vi "Main.vi"() -> ()   [LabVIEW 2017]
uses:
  GlobalFlash.vi
panel:
  out "?":dbl(slide) scale=0.0..100.0
  in  "Enable Alarm 7":bool=TRUE
  in  "Enable Alarm 6":bool=TRUE
  in  "Sensor 5":dbl(slide) scale=0.0..100.0
  out "Enable Alarm 5":u32(colorbox)=350218
  in  "Enable Alarm 5":bool
  in  "Sensor 4":dbl(slide) scale=0.0..100.0
  out "Enable Alarm 4":u32(colorbox)=350218
  in  "Enable Alarm 4":bool
  in  "Sensor 3":dbl(slide) scale=0.0..100.0
  out "?":u32(colorbox)=350218
  in  "Enable Alarm 3":bool
  out "?":u32(colorbox)=350218
  in  "Enable Alarm 2":bool
  in  "Sensor 2":dbl(slide) scale=0.0..100.0
  out "?":u32(colorbox)=350218
  in  "Reset1":bool
  in  "Reset2":bool
  in  "Reset3":bool
  in  "Reset4":bool
  in  "Reset5":bool
  in  "Enable Alarm 1":bool
  in  "Sensor 1":dbl(slide) scale=0.0..100.0
  # "°c"
  # "Management"
  # "Self test"
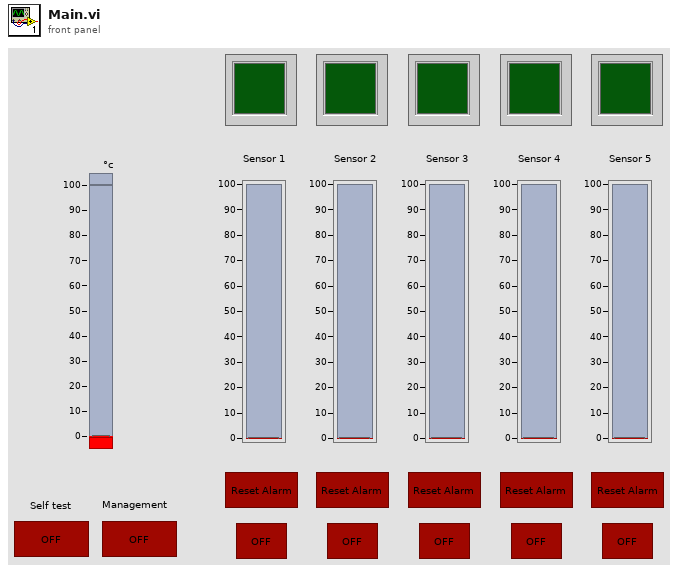
[diagram p1: front panel]
types:
  T1 = enum8{"Enabled", "Disabled", "Disabled and Grayed Out"}
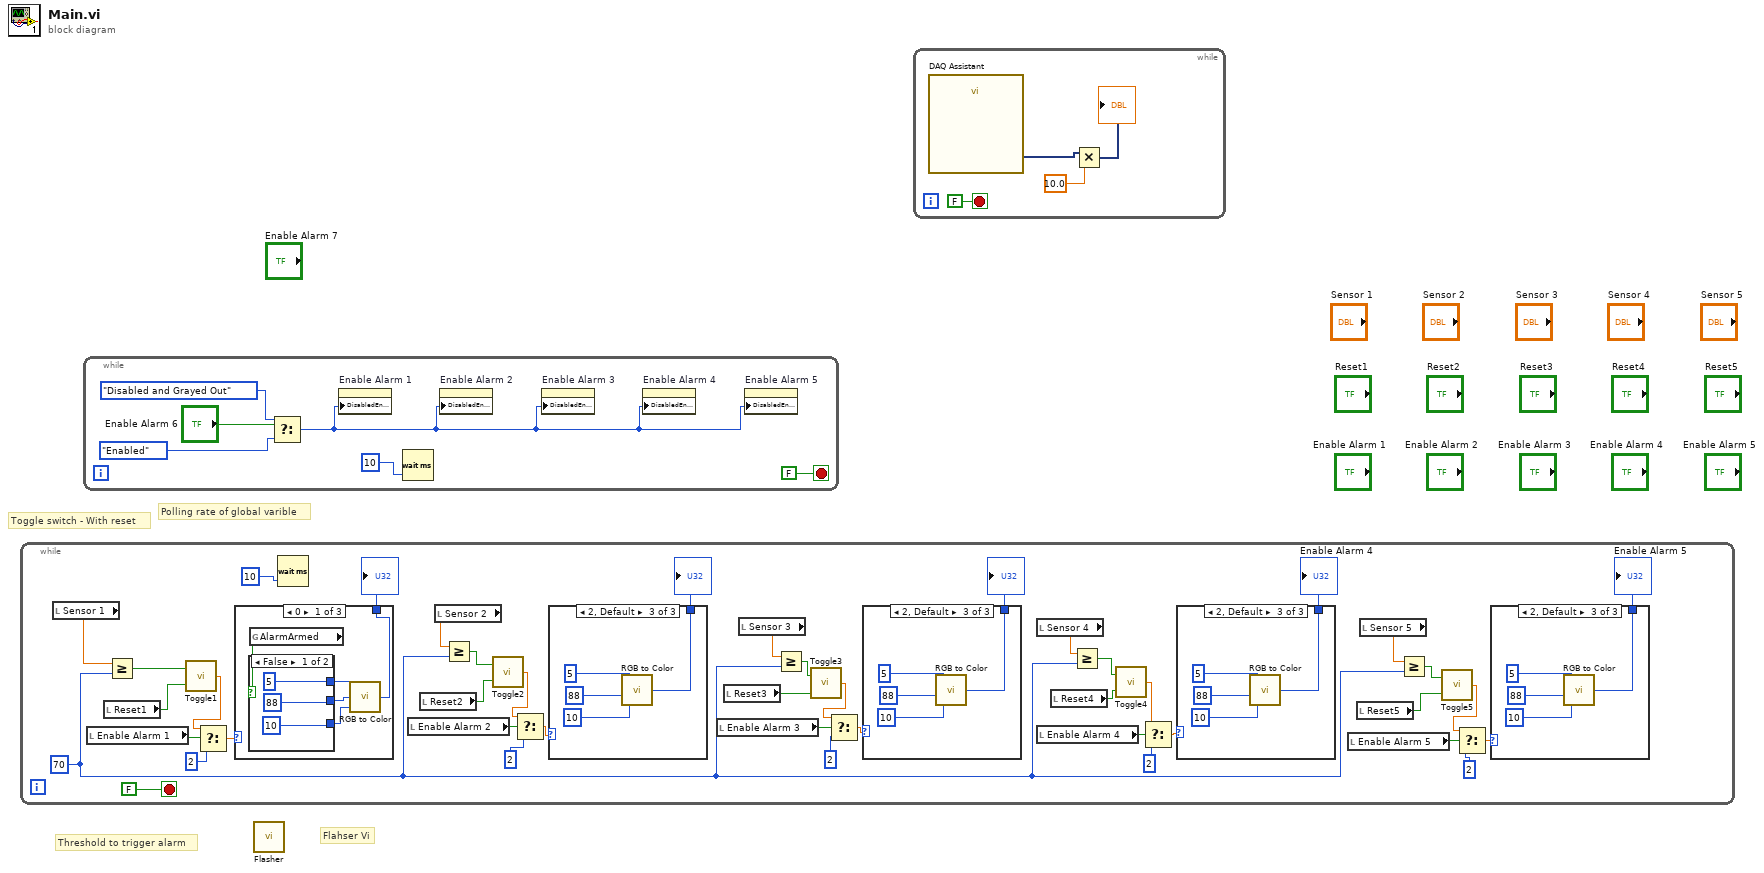
[diagram p0: block diagram]
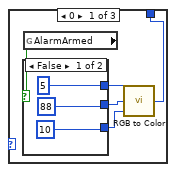
[diagram p2: hidden frame]
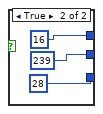
[diagram p3: hidden frame]
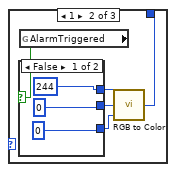
[diagram p4: hidden frame]
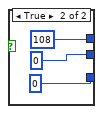
[diagram p5: hidden frame]
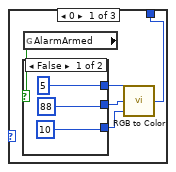
[diagram p6: hidden frame]
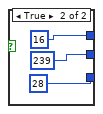
[diagram p7: hidden frame]
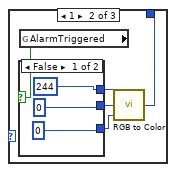
[diagram p8: hidden frame]
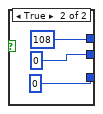
[diagram p9: hidden frame]
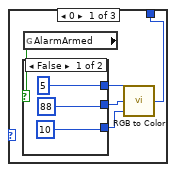
[diagram p10: hidden frame]
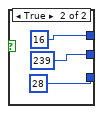
[diagram p11: hidden frame]
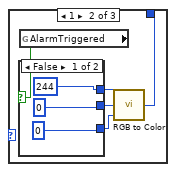
[diagram p12: hidden frame]
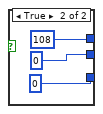
[diagram p13: hidden frame]
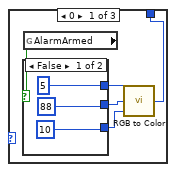
[diagram p14: hidden frame]
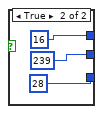
[diagram p15: hidden frame]
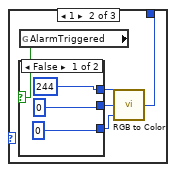
[diagram p16: hidden frame]
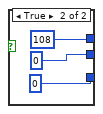
[diagram p17: hidden frame]
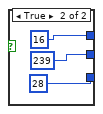
[diagram p18: hidden frame]
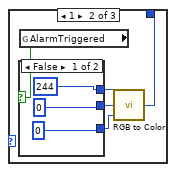
[diagram p19: hidden frame]
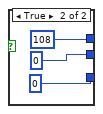
[diagram p20: hidden frame]
diagram:
  # "Toggle switch - With reset"
  # "Flahser Vi"
  # "Polling rate of global varible"
  # "Threshold to trigger alarm"
  n1 = while {
    stop <- FALSE stop-if-true
    w16 = 70
    n2 = local read "Sensor 1"() -> (w24:dbl)
    n3 = local read "Enable Alarm 1"() -> (w22:bool)
    n4 = local read "Reset1"() -> (w9:bool)
    n5 = Greater Or Equal?(x=w24, y=w16) -> (x >= y?=w7:bool)
    n6 = call "Toggle1.vi"("Boolean 2"=w9, "Boolean"=w7) -> ("Numeric"=w8:dbl)
    n7 = Select(t=w8, s=w22, f=2) -> (s? t:f=w23:dbl)
    n8 = case shown="0" w23 {
      tunnel: [w149 w159 w173] -> w41
      frame 0 {
        n9 = global read "GlobalFlash.vi" "AlarmArmed"() -> (w152:bool)
        n10 = case shown="False" w152 {
          tunnel: [10 28] -> w151
          tunnel: [88 239] -> w150
          tunnel: [5 16] -> w148
          frame False {
          }
          frame True {
          }
        }
        n11 = call <vilib>:"RGB to Color.vi"("B"=w151, "G"=w150, "R"=w148) -> ("Color"=w149:u32)
      }
      frame 1 {
        n12 = global read "GlobalFlash.vi" "AlarmTriggered"() -> (w161:bool)
        n13 = case shown="False" w161 {
          tunnel: [0 0] -> w163
          tunnel: [0 0] -> w162
          tunnel: [244 108] -> w160
          frame False {
          }
          frame True {
          }
        }
        n14 = call <vilib>:"RGB to Color.vi"("B"=w163, "G"=w162, "R"=w160) -> ("Color"=w159:u32)
      }
      frame 2, Default {
        n15 = call <vilib>:"RGB to Color.vi"("B"=10, "G"=88, "R"=5) -> ("Color"=w173:u32)
      }
    }
    "?" <- w41
    n16 = Wait (ms)(milliseconds to wait=10) -> ()  [unwired: 1 out]
    n17 = local read "Enable Alarm 2"() -> (w33:bool)
    n18 = local read "Reset2"() -> (w14:bool)
    n19 = local read "Sensor 2"() -> (w40:dbl)
    n20 = Greater Or Equal?(x=w40, y=w16) -> (x >= y?=w15:bool)
    n21 = call "Toggle2.vi"("Boolean 2"=w14, "Boolean"=w15) -> ("Numeric"=w13:dbl)
    n22 = Select(t=w13, s=w33, f=2) -> (s? t:f=w32:dbl)
    n23 = case shown="2, Default" w32 {
      tunnel: [w123 w133 w147] -> w39
      frame 0 {
        n24 = global read "GlobalFlash.vi" "AlarmArmed"() -> (w126:bool)
        n25 = case shown="False" w126 {
          tunnel: [10 28] -> w125
          tunnel: [88 239] -> w124
          tunnel: [5 16] -> w122
          frame False {
          }
          frame True {
          }
        }
        n26 = call <vilib>:"RGB to Color.vi"("B"=w125, "G"=w124, "R"=w122) -> ("Color"=w123:u32)
      }
      frame 1 {
        n27 = global read "GlobalFlash.vi" "AlarmTriggered"() -> (w135:bool)
        n28 = case shown="False" w135 {
          tunnel: [0 0] -> w137
          tunnel: [0 0] -> w136
          tunnel: [244 108] -> w134
          frame False {
          }
          frame True {
          }
        }
        n29 = call <vilib>:"RGB to Color.vi"("B"=w137, "G"=w136, "R"=w134) -> ("Color"=w133:u32)
      }
      frame 2, Default {
        n30 = call <vilib>:"RGB to Color.vi"("B"=10, "G"=88, "R"=5) -> ("Color"=w147:u32)
      }
    }
    "?" <- w39
    n31 = local read "Enable Alarm 3"() -> (w18:bool)
    n32 = local read "Reset3"() -> (w11:bool)
    n33 = local read "Sensor 3"() -> (w17:dbl)
    n34 = Greater Or Equal?(x=w17, y=w16) -> (x >= y?=w12:bool)
    n35 = call "Toggle3.vi"("Boolean 2"=w11, "Boolean"=w12) -> ("Numeric"=w10:dbl)
    n36 = Select(t=w10, s=w18, f=2) -> (s? t:f=w20:dbl)
    n37 = case shown="2, Default" w20 {
      tunnel: [w97 w107 w121] -> w38
      frame 0 {
        n38 = global read "GlobalFlash.vi" "AlarmArmed"() -> (w100:bool)
        n39 = case shown="False" w100 {
          tunnel: [10 28] -> w99
          tunnel: [88 239] -> w98
          tunnel: [5 16] -> w96
          frame False {
          }
          frame True {
          }
        }
        n40 = call <vilib>:"RGB to Color.vi"("B"=w99, "G"=w98, "R"=w96) -> ("Color"=w97:u32)
      }
      frame 1 {
        n41 = global read "GlobalFlash.vi" "AlarmTriggered"() -> (w109:bool)
        n42 = case shown="False" w109 {
          tunnel: [0 0] -> w111
          tunnel: [0 0] -> w110
          tunnel: [244 108] -> w108
          frame False {
          }
          frame True {
          }
        }
        n43 = call <vilib>:"RGB to Color.vi"("B"=w111, "G"=w110, "R"=w108) -> ("Color"=w107:u32)
      }
      frame 2, Default {
        n44 = call <vilib>:"RGB to Color.vi"("B"=10, "G"=88, "R"=5) -> ("Color"=w121:u32)
      }
    }
    "?" <- w38
    n45 = local read "Sensor 4"() -> (w37:dbl)
    n46 = local read "Enable Alarm 4"() -> (w30:bool)
    n47 = local read "Reset4"() -> (w5:bool)
    n48 = Greater Or Equal?(x=w37, y=w16) -> (x >= y?=w6:bool)
    n49 = call "Toggle4.vi"("Boolean 2"=w5, "Boolean"=w6) -> ("Numeric"=w4:dbl)
    n50 = Select(t=w4, s=w30, f=2) -> (s? t:f=w31:dbl)
    n51 = case shown="2, Default" w31 {
      tunnel: [w71 w81 w95] -> w36
      frame 0 {
        n52 = global read "GlobalFlash.vi" "AlarmArmed"() -> (w74:bool)
        n53 = case shown="False" w74 {
          tunnel: [10 28] -> w73
          tunnel: [88 239] -> w72
          tunnel: [5 16] -> w70
          frame False {
          }
          frame True {
          }
        }
        n54 = call <vilib>:"RGB to Color.vi"("B"=w73, "G"=w72, "R"=w70) -> ("Color"=w71:u32)
      }
      frame 1 {
        n55 = global read "GlobalFlash.vi" "AlarmTriggered"() -> (w83:bool)
        n56 = case shown="False" w83 {
          tunnel: [0 0] -> w85
          tunnel: [0 0] -> w84
          tunnel: [244 108] -> w82
          frame False {
          }
          frame True {
          }
        }
        n57 = call <vilib>:"RGB to Color.vi"("B"=w85, "G"=w84, "R"=w82) -> ("Color"=w81:u32)
      }
      frame 2, Default {
        n58 = call <vilib>:"RGB to Color.vi"("B"=10, "G"=88, "R"=5) -> ("Color"=w95:u32)
      }
    }
    "Enable Alarm 4" <- w36
    n59 = local read "Enable Alarm 5"() -> (w29:bool)
    n60 = local read "Reset5"() -> (w3:bool)
    n61 = local read "Sensor 5"() -> (w35:dbl)
    n62 = Greater Or Equal?(x=w35, y=w16) -> (x >= y?=w2:bool)
    n63 = call "Toggle5.vi"("Boolean 2"=w3, "Boolean"=w2) -> ("Numeric"=w1:dbl)
    n64 = Select(t=w1, s=w29, f=2) -> (s? t:f=w28:dbl)
    n65 = case shown="2, Default" w28 {
      tunnel: [w45 w55 w69] -> w34
      frame 0 {
        n66 = global read "GlobalFlash.vi" "AlarmArmed"() -> (w48:bool)
        n67 = case shown="False" w48 {
          tunnel: [10 28] -> w47
          tunnel: [88 239] -> w46
          tunnel: [5 16] -> w44
          frame False {
          }
          frame True {
          }
        }
        n68 = call <vilib>:"RGB to Color.vi"("B"=w47, "G"=w46, "R"=w44) -> ("Color"=w45:u32)
      }
      frame 1 {
        n69 = global read "GlobalFlash.vi" "AlarmTriggered"() -> (w57:bool)
        n70 = case shown="False" w57 {
          tunnel: [0 0] -> w59
          tunnel: [0 0] -> w58
          tunnel: [244 108] -> w56
          frame False {
          }
          frame True {
          }
        }
        n71 = call <vilib>:"RGB to Color.vi"("B"=w59, "G"=w58, "R"=w56) -> ("Color"=w55:u32)
      }
      frame 2, Default {
        n72 = call <vilib>:"RGB to Color.vi"("B"=10, "G"=88, "R"=5) -> ("Color"=w69:u32)
      }
    }
    "Enable Alarm 5" <- w34
  }
  n73 = while {
    stop <- FALSE stop-if-true
    n74 = Select(t=T1."Disabled and Grayed Out" ("Disabled"), s="Enable Alarm 6", f=T1."Enabled" ("Disabled")) -> (s? t:f=w178:T1)
    n75 = property on="Enable Alarm 1" class="Bool (strict)"("DisabledEnum"=w178) -> ()  [unwired: 2 in, 2 out]
    n76 = Wait (ms)(milliseconds to wait=10) -> ()  [unwired: 1 out]
    n77 = property on="Enable Alarm 2" class="Bool (strict)"("DisabledEnum"=w178) -> ()  [unwired: 2 in, 2 out]
    n78 = property on="Enable Alarm 3" class="Bool (strict)"("DisabledEnum"=w178) -> ()  [unwired: 2 in, 2 out]
    n79 = property on="Enable Alarm 4" class="Bool (strict)"("DisabledEnum"=w178) -> ()  [unwired: 2 in, 2 out]
    n80 = property on="Enable Alarm 5" class="Bool (strict)"("DisabledEnum"=w178) -> ()  [unwired: 2 in, 2 out]
  }
  n81 = call "Flasher.vi"() -> ()  [unwired: 12 in]
  n82 = while {
    stop <- FALSE stop-if-true
    n83 = call "DAQ Assistant"() -> ("data"=w181:dynamicdata)  [unwired: 16 in, 3 out]
    n84 = Multiply(x=w181, y=10.0) -> (x*y=→"?":dynamicdata)
  }
